vi "Run Servicer.vi"() -> ()   [LabVIEW 2019, in "gRPC-servicer.lvlib" / "Servicer.lvclass"]
uses:
  Servicer.lvclass
  ServiceBase/ServiceBase.lvclass
panel:
  in  "Async [T] / Sync [F]":bool
  out "Listening Port":i32
  in  "Stop":bool
  in  "Server Address":string="localhost:50051"
  in  "Server Certificate File (.crt)":path
  in  "Server Key File (.key)":path
  # "Note: If you want the service to auto find the listening port, then enter the port number in \"Server Address\" as 0. Ex: localhost:0"
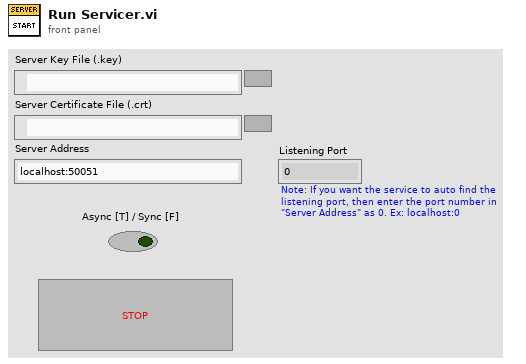
[diagram p1: front panel]
types:
  T1 = typedef "grpc-lvsupport.lvlib/grpcId.ctl" = u64
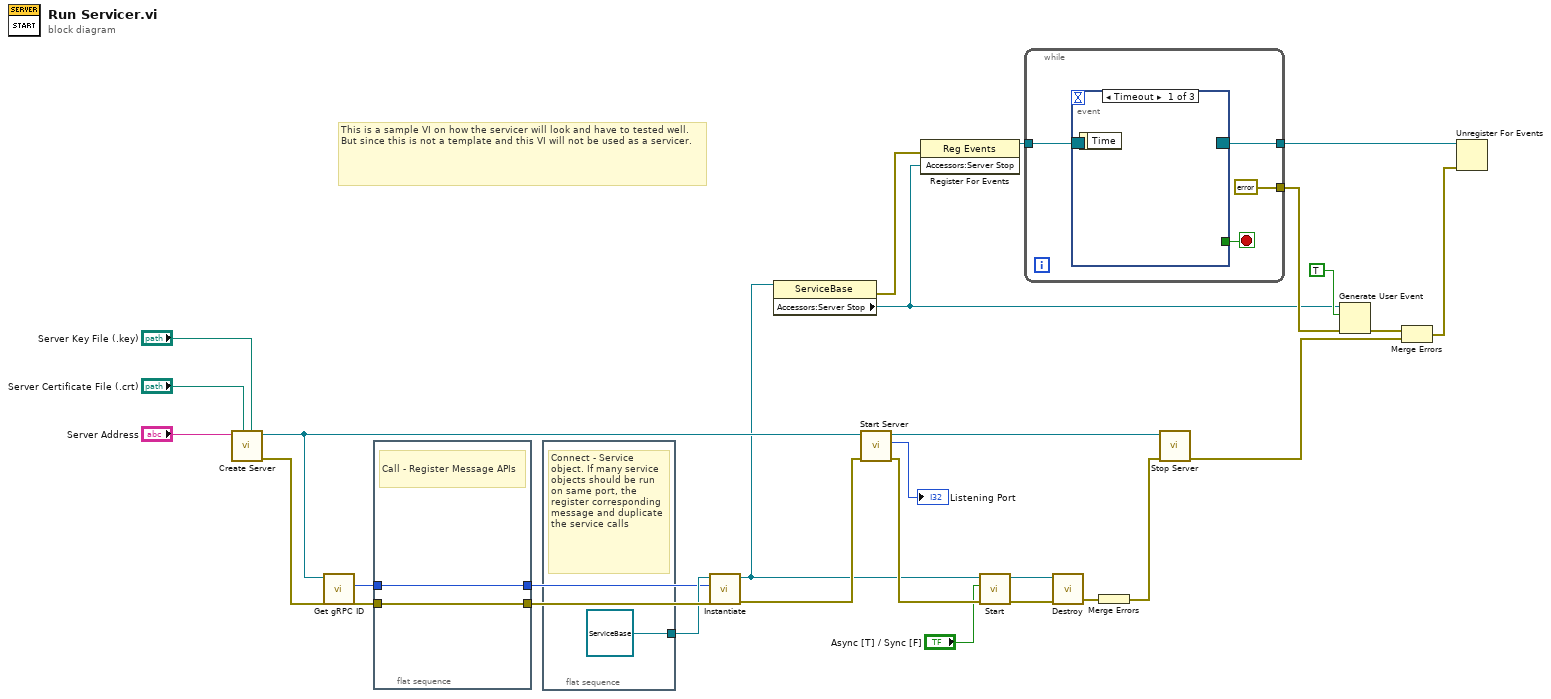
[diagram p0: block diagram]
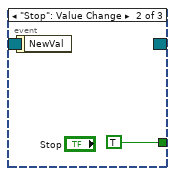
[diagram p2: hidden frame]
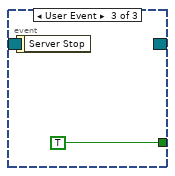
[diagram p3: hidden frame]
diagram:
  # "This is a sample VI on how the servicer will look and have to tested well. But since this is not a template and this VI will not be used as a servicer."
  n1 = call "Create Server.vi"("Server Key File (.key)"="Server Key File (.key)", "Server Certificate File (.crt)"="Server Certificate File (.crt)", "Server Address"="Server Address") -> ("error out"=w20:errorcluster, "gRPC server out"=w9:refnum<class "Servicer.lvclass">)  [unwired: 7 in]
  n2 = call "Get gRPC ID.vi"("gRPC server in"=w9) -> ("gRPC ID"=w5:T1)  [unwired: 9 in, 1 out]
  n3 = flat-sequence {
    tunnel: w5 -> [w29]
    tunnel: w20 -> [w30]
    tunnel: [w30] -> w19
    tunnel: [w29] -> w4
    frame #0 {
      # "Call - Register Message APIs"
    }
  }
  n4 = flat-sequence {
    tunnel: [refnum<class "ServiceBase.lvclass"> refnum ("gRPC-servicer.lvlib:iService.lvclass")] -> w6
    frame #0 {
      # "Connect - Service object. If many service objects should be run on same port, the register corresponding message and duplicate the service calls"
    }
  }
  n5 = call-dynamic "Instantiate.vi"("error in"=w19, "gRPCid"=w4, "gRPC service in"=w6) -> ("error out"=w27:errorcluster, "gRPC service out"=w1:refnum<class "ServiceBase.lvclass">)  [unwired: 7 in]
  n6 = property class="ServiceBase"(reference=w1) -> (error out=w28:errorcluster, "Accessors:Server Stop"=w7:refnum<user-event>)  [unwired: 1 in, 1 out]
  n7 = call "Start Server.vi"("error in"=w27, "gRPC server in"=w9) -> ("error out"=w18:errorcluster, "Listening Port"=→"Listening Port":i32, "gRPC server out"=w16:refnum<class "Servicer.lvclass">)  [unwired: 7 in]
  n8 = register-events(error in=w28, w7) -> (reference out=w12:refnum<event-registration>)  [unwired: 1 in, 1 out]
  n9 = call-dynamic "Start.vi"("error in"=w18, "ASync [T]"="Async [T] / Sync [F]", "gRPC service in"=w1) -> ("error out"=w17:errorcluster, "gRPC service out"=w3:refnum<class "ServiceBase.lvclass">)  [unwired: 7 in]
  n10 = while {
    tunnel: w12 -> [w34]
    tunnel: [w32] -> w11
    tunnel: [errorcluster {"status"=FALSE, "code"=0, "source"=""} ("error constant")] -> w22
    stop <- w33 stop-if-true
    n11 = event shown="[0] Timeout" {
      selector: w34 -> [_ _ _]
      dyn-events: [_ _ _] -> w32
      timeout: _ -> [_ _ _]
      tunnel: [_ TRUE TRUE] -> w33
      event Timeout {
        n12 = event-data() -> ()  [unwired: 1 in, 1 out]
      }
      event "Stop": Value Change {
        n13 = event-data() -> ()  [unwired: 1 in, 1 out]
      }
      event User Event {
        n14 = event-data() -> ()  [unwired: 1 in, 1 out]
      }
    }
  }
  n15 = call-dynamic "Destroy.vi"("error in"=w17, "gRPC service in"=w3) -> ("error out"=w26:errorcluster)  [unwired: 8 in, 1 out]
  n16 = Merge Errors(w26) -> (w25:errorcluster)
  n17 = call "Stop Server.vi"("error in"=w25, "gRPC server in"=w16) -> ("error out"=w21:errorcluster)  [unwired: 9 in]
  n18 = Generate User Event(user event=w7, event data cluster=TRUE ("event data"), error in=w22) -> (error out=w24:errorcluster)  [unwired: 1 in, 1 out]
  n19 = Merge Errors(w24, w21) -> (w23:errorcluster)
  n20 = Unregister For Events(event registration refnum=w11, error in=w23) -> ()  [unwired: 1 out]
